vi "Setup.vi"(8 "Error In":errorcluster) -> (0 "Error Out":errorcluster, 3 "lv-libssh2 Shared Library":path)   [LabVIEW 2018, in "Tests.lvlib" / "SFTP Attributes.lvlib"]
uses:
  SFTP Attributes.lvlib
  src/Toolkit/Toolkit.lvlib
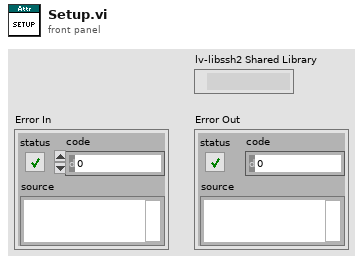
[diagram p1: front panel]
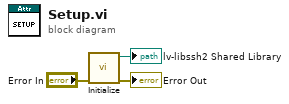
[diagram p0: block diagram]
diagram:
  n1 = call "Initialize.vi"("Error In"="Error In") -> ("Error Out"=→"Error Out":errorcluster, "lv-libssh2 Shared Library Out"=→"lv-libssh2 Shared Library":path)  [unwired: 9 in]
